vi "Cleanup.vi"(8 "error in (no error)":errorcluster, 11 "PanelArray in":refnum<class "ArrayManager.lvclass">) -> (0 "error out":errorcluster)   [LabVIEW 2020, in "OOPanel.lvlib" / "ArrayManager.lvclass"]
uses:
  ArrayManager.lvclass
  ArrayManager.lvclass/ArrayManager.ctl
  Manager/Manager.lvclass
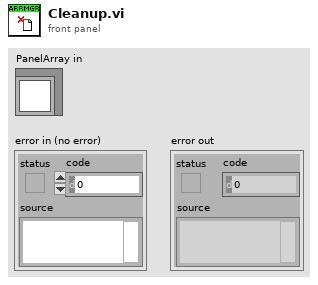
[diagram p1: front panel]
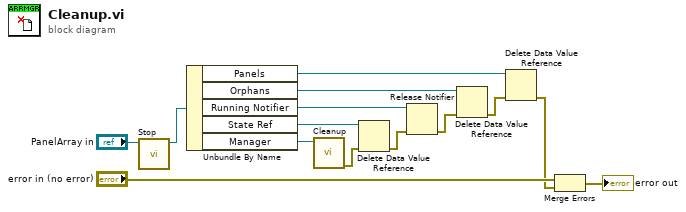
[diagram p0: block diagram]
diagram:
  n1 = call "Stop.vi"("ArrayManager in"="PanelArray in") -> ("ArrayManager out"=w10:refnum<class "ArrayManager.lvclass">)  [unwired: 9 in, 1 out]
  n2 = Unbundle By Name(w10) -> ("Panels"=w4:refnum<data-value>, "Orphans"=w5:refnum<data-value>, "Running Notifier"=w7:refnum<notifier>, "State Ref"=w9:refnum<data-value>, "Manager"=w13:refnum<class "Manager.lvclass">)
  n3 = call "Cleanup.vi"("Manager in"=w13) -> ("error out"=w8:errorcluster)  [unwired: 10 in]
  n4 = Delete Data Value Reference(data value reference=w9, error in=w8) -> (error out=w6:errorcluster)  [unwired: 1 out]
  n5 = Release Notifier(notifier=w7, error in (no error)=w6) -> (error out=w3:errorcluster)  [unwired: 1 in, 2 out]
  n6 = Delete Data Value Reference(data value reference=w5, error in=w3) -> (error out=w2:errorcluster)  [unwired: 1 out]
  n7 = Delete Data Value Reference(data value reference=w4, error in=w2) -> (error out=w1:errorcluster)  [unwired: 1 out]
  n8 = Merge Errors("error in (no error)", w1) -> (→"error out":errorcluster)
